vi "ampltude_modifier_for_ramp.vi"(8 "readout iter i":dbl, 9 "no. ramping ROPPs":dbl, 11 "orig waveform":waveform(dbl)) -> (3 "amplitude modulated waveform":waveform(dbl))   [LabVIEW 2019]
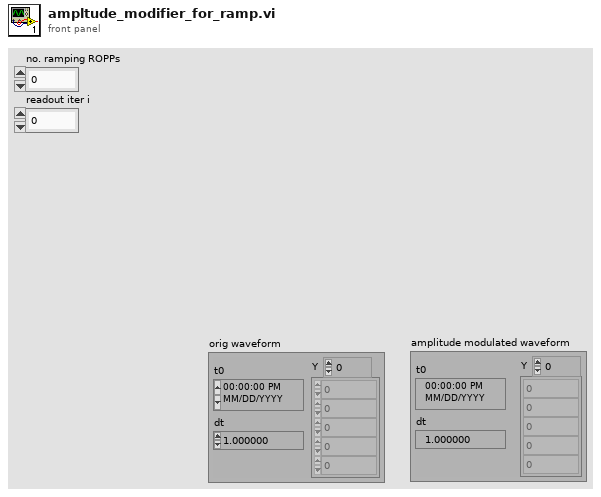
[diagram p1: front panel]
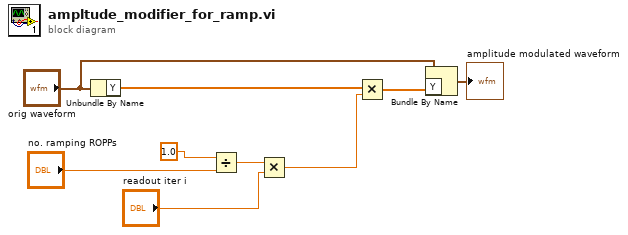
[diagram p0: block diagram]
diagram:
  n1 = Unbundle By Name("orig waveform") -> ("Y"=w4:dbl[])
  n2 = Divide(x=1.0 ("end"), y="no. ramping ROPPs") -> (x/y=w9:dbl)
  n3 = Multiply(x=w9, y="readout iter i") -> (x*y=w5:dbl)
  n4 = Multiply(x=w4, y=w5) -> (x*y=w3:dbl[])
  n5 = Bundle By Name(cluster="orig waveform", "Y"=w3) -> (→"amplitude modulated waveform":waveform(dbl))
